vi "LQR_CLEst.vi"() -> ()   [LabVIEW 2019]
uses:
  <vilib>/Analysis/Matrix/Datatypes/RealMatrix.ctl
  <vilib>/Platform/TimedLoop/XDataNode/timing_clust.ctl
  <vilib>/Platform/TimedLoop/XDataNode/nitl_modes.ctl
  <vilib>/Platform/TimedLoop/XDataNode/wakeup.ctl
  <vilib>/Simulation/Shared/_Datatypes/SIM SISO Transfer Function.ctl
  <vilib>/myRIO/Instrument Drivers/Onboard IO/AI/typedefs/AI Reference.ctl
  <vilib>/myRIO/Common/Instrument Driver Framework/Utilities/typedefs/myRIO Generic Hardware Reference.ctl
  <vilib>/myRIO/Common/Instrument Driver Framework/Utilities/typedefs/Hardware Version Enum.ctl
  <vilib>/myRIO/Common/Instrument Driver Framework/Utilities/typedefs/myRIO v1.0 Reference.ctl
  <vilib>/myRIO/Common/Instrument Driver Framework/Utilities/typedefs/Generic FPGA Reference.ctl
  <vilib>/myRIO/Common/Instrument Driver Framework/myRIO v1.0/AI/typedefs/AI Channels List.ctl
  <vilib>/myRIO/Common/Instrument Driver Framework/myRIO v1.0/AI/typedefs/AI Channels Enum.ctl
  <vilib>/myRIO/Common/Instrument Driver Framework/Utilities/typedefs/Analog Scaling Constants List.ctl
  <vilib>/myRIO/Common/Instrument Driver Framework/Utilities/typedefs/Analog Scaling Constants.ctl
  <vilib>/userDefined/High Color/nirio_resource_hc.ctl
  <vilib>/myRIO/Instrument Drivers/Onboard IO/AO/typedefs/AO Reference.ctl
  <vilib>/myRIO/Common/Instrument Driver Framework/myRIO v1.0/AO/typedefs/AO Channels List.ctl
  <vilib>/myRIO/Common/Instrument Driver Framework/myRIO v1.0/AO/typedefs/AO Channels Enum.ctl
  <vilib>/myRIO/Common/Instrument Driver Framework/Utilities/vis/Is FPGA Ref Available.vi
  <vilib>/myRIO/Common/Instrument Driver Framework/myRIO v1.0/AI/vis/myRIO v1.1 Open AI.vi
  <vilib>/myRIO/Instrument Drivers/Onboard IO/AI/vis/Read.vi
  <vilib>/Simulation/DiscreteLinear/Implementation/NILVSim Discrete Transfer Function Direct.llb/SIM Discrete Transfer Function Diagram (SISO).vi
  <vilib>/myRIO/Common/Instrument Driver Framework/myRIO v1.0/AO/vis/myRIO v1.1 Open AO.vi
  <vilib>/myRIO/Instrument Drivers/Onboard IO/AO/vis/Write.vi
  <vilib>/myRIO/Common/Instrument Driver Framework/Utilities/vis/Validate Channels.vi
  <vilib>/myRIO/Common/Instrument Driver Framework/myRIO v1.0/AI/vis/myRIO v1.0 Reserve AI.vi
  <vilib>/Simulation/ContinuousLinear/Implementation/Shared/SIM Transfer Function Support.llb/SIM TransferFunction Normalize to Buffer.vi
  <vilib>/Simulation/DiscreteLinear/Implementation/Shared/SIM Init Discrete States.vi
  <vilib>/Simulation/DiscreteLinear/Implementation/NILVSim Discrete Transfer Function Direct.llb/SIM Transfer Function Direct core (SISO).vi
  <vilib>/myRIO/Common/Instrument Driver Framework/myRIO v1.0/AO/vis/myRIO v1.0 Reserve AO.vi
  <vilib>/myRIO/Common/Instrument Driver Framework/myRIO v1.0/AI/vis/myRIO v1.0 Build MUX Configuration AI.vi
  <vilib>/myRIO/Common/Instrument Driver Framework/myRIO v1.0/Resource Manager/vis/myRIO v1.0 Reserve Channel List.vi
  <vilib>/Simulation/ContinuousLinear/Implementation/Shared/SIM Transfer Function Support.llb/SIM TransferFunction Normalize.vi
  <vilib>/myRIO/Common/Instrument Driver Framework/myRIO v1.0/AO/vis/myRIO v1.0 Build MUX Configuration AO.vi
  <vilib>/myRIO/Common/Instrument Driver Framework/myRIO v1.0/Resource Manager/vis/myRIO v1.0 Reserve Channel.vi
  <vilib>/myRIO/Common/Instrument Driver Framework/myRIO v1.0/Resource Manager/vis/myRIO v1.0 Unreserve Channel.vi
  <vilib>/Simulation/Implementation/Shared/SIM Polynomials.llb/SIM Remove Zero Coefficients (DBL).vi
  <vilib>/myRIO/Common/Instrument Driver Framework/myRIO v1.0/Resource Manager/vis/myRIO v1.0 Build Mutex Name.vi
  <vilib>/Simulation/Implementation/Shared/SIM Polynomials.llb/SIM Divide Polynomials (DBL).vi
  <vilib>/Simulation/Implementation/Shared/SIM BuildSimErr.vi
  <vilib>/Utility/VariantDataType/GetNumericInfo.vi
  <vilib>/Utility/error.llb/Error Cluster From Error Code.vi
  <vilib>/myRIO/Common/Instrument Driver Framework/myRIO v1.0/myRIO v1.1 Open.vi
  <vilib>/myRIO/Common/Instrument Driver Framework/myRIO v1.0/AI/vis/myRIO v1.0 Get Scaling Constants AI.vi
  <vilib>/myRIO/Common/Instrument Driver Framework/Utilities/vis/IO Manager.vi
  <vilib>/myRIO/Common/Instrument Driver Framework/Utilities/vis/Configuration Manager.vi
  <vilib>/myRIO/Common/Instrument Driver Framework/myRIO v1.0/myRIO v1.0 Close.vi
  <vilib>/myRIO/Common/Instrument Driver Framework/myRIO v1.0/AI/vis/myRIO v1.0 Read AI.vi
  <vilib>/myRIO/Common/Instrument Driver Framework/myRIO v1.0/AO/vis/myRIO v1.0 Get Scaling Constants AO.vi
  <vilib>/myRIO/Common/Instrument Driver Framework/myRIO v1.0/AO/vis/myRIO v1.0 Write AO.vi
  <vilib>/Analysis/Matrix/Numeric/Multiply/Multiply - RM,RM.vi
  <vilib>/Analysis/Matrix/Numeric/Subtract/Subtract (Elementwise) - R,RM.vi
  <vilib>/Analysis/Matrix/Numeric/Multiply/Multiply - RM,R.vi
  <vilib>/Analysis/Matrix/Numeric/Add/Add - RM,RM.vi
  <vilib>/platform/TimedLoop/XDataNode/XDataNode.xnode
  <vilib>/Simulation/Implementation/XNodeFramework/SimXNode/SimX.xnode
  <vilib>/myRIO/Express VI/Onboard IO/AI/AI Express VI.xnode
  <vilib>/myRIO/Instrument Drivers/Onboard IO/AI/vis/myRIO AI Open.xnode
  <vilib>/myRIO/Express VI/Onboard IO/AO/AO Express VI.xnode
  <vilib>/myRIO/Instrument Drivers/Onboard IO/AO/vis/myRIO AO Open.xnode
  <vilib>/Platform/TimedLoop/XDataNode/XDNodeRunTimeDep.lvlib
  <vilib>/myRIO/Instrument Drivers/Onboard IO/AI/AI.lvlib
  <vilib>/myRIO/Instrument Drivers/Onboard IO/AO/AO.lvlib
  <vilib>/ptbypt/NI_PtbyPt.lvlib
  <vilib>/Analysis/Matrix/NI_Matrix.lvlib
panel:
  in  "amplitude":dbl=1.0 format="%0.2f"
  out "Impulse Pattern":dbl(graph)
  out "output y(k)":dbl=6.43996164946016e-05
  in  "D":dbl=7.3
  in  "P":dbl=5291.0
  out "x*y":dbl(graph)=-8.32082689025263
  in  "C":T1=[[1.0, 0.0]]
  out "transposed matrix":T1=[[7.6247197208905344e-06], [0.00010412510161981911]]
  in  "B":T1=[[0.0], [17.2685]]
  in  "A":T1=[[0.0, 1.0], [-5529.8, -0.5327]]
  in  "L":T1=[[2200.0], [1953300.0]]
  in  "stopNoise":bool=TRUE
  in  "gain_noise":dbl=0.2
  out "uniform white noise":dbl(graph)=-0.031193239239623867
  in  "AmpWhitehNoise":dbl=1.0 format="%0.2f"
  out "Iteration Duration":i64(graph)=347
  in  "Max FRF current 0-1000mA":dbl=4.0
  in  "Stop FRF":bool=TRUE
  in  "esc":bool
  out "x[um]":cluster{dbl, dbl, dbl, dbl, dbl}(graph)={-8.303163599999976, 0.03990822535355048, -0.0, -8.32082689025263, 946.4168275057085}
  out "Current Output EM":dbl(graph)=0.03990822535355048
  in  "Stop EM + FRF":bool=TRUE
  out "left[V]":dbl=-0.0
  out "right[V]":dbl=-0.0
  out "um":dbl=376.9531636
  # "mA"
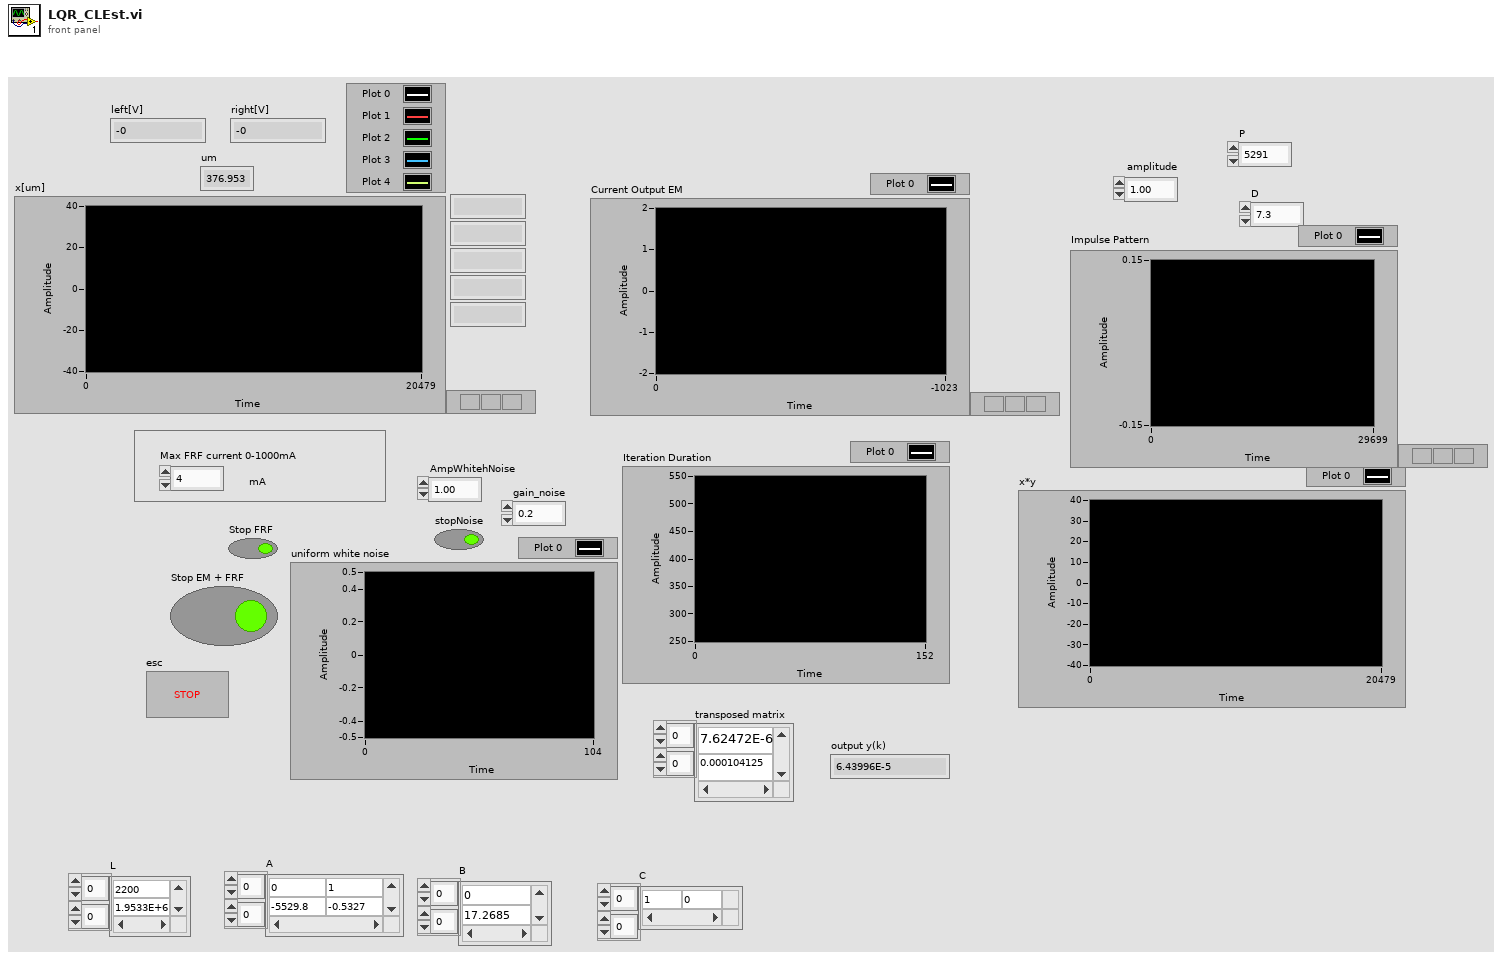
[diagram p1: front panel]
types:
  T1 = typedef "NI_Matrix.lvlib/RealMatrix.ctl" = dbl[][]
  T2 = typedef "XDNodeRunTimeDep.lvlib/timing_clust.ctl" = cluster{"Expected End [f-1]":u64, "Actual End [f-1]":u64, "Finished Late? [f-1]":bool, "Expected End [i-1]":u64, "Actual End [i-1]":u64, "Finished Late? [i-1]":bool, "Expected Start [i]":u64, "Actual Start [i]":u64, "Expected Start [f]":u64, "Actual Start [f]":u64, "Source Name":string, "Structure Name":string, "Period":i64, "Deadline":i64, "Offset":i64, "Start":i64, "Priority":i32, "Timeout":i32, "Mode":T3, "Wakeup Reason":T4, "Error":errorcluster, "Source Type":string, "Secondary Source Type":string, "Global End Time":u64, "Global Start Time":u64, "Frame Duration":u64, "Iteration Duration":u64, "Assigned CPU":i32, "I/O Scan Engine Mode":u32}
  T3 = typedef "XDNodeRunTimeDep.lvlib/nitl_modes.ctl" = enum32{"No Change", "Process missed periods, maintain original phase", "Discard missed periods, maintain original phase", "Process missed periods, ignore original phase", "Discard missed periods, ignore original phase"}
  T4 = typedef "XDNodeRunTimeDep.lvlib/wakeup.ctl" = enum32{"Normal", "Aborted", "Asynchronous wakeup", "Timing source error", "Timed loop error", "Timeout"}
  T5 = typedef "SIM SISO Transfer Function.ctl" = cluster{"Numerator":dbl[], "Denominator":dbl[]}
  T6 = typedef "AI.lvlib/AI Reference.ctl" = cluster{"myRIO Reference":T7, "AI Channels List":T11, "AI Scaling Constants List":T13}
  T7 = typedef "myRIO Generic Hardware Reference.ctl" = cluster{"myRIO Model":T8, "myRIO Hardware Reference":T9}
  T8 = typedef "Hardware Version Enum.ctl" = enum16{"Unknown", "myRIO-1900", "myRIO-1950", "roboRIO", "NI ELVIS RIO CM", "ELVIS III"}
  T9 = typedef "myRIO v1.0 Reference.ctl" = cluster{"Generic FPGA Reference":T10, "Allow multiple opens":bool}
  T10 = typedef "Generic FPGA Reference.ctl" = refnum<k20>
  T11 = typedef "AI Channels List.ctl" = T12[]
  T12 = typedef "AI Channels Enum.ctl" = enum16{"Not Connected", "AudioIn/Left", "AudioIn/Right", "C/AI0", "C/AI1", "A/AI0", "A/AI1", "A/AI2", "A/AI3", "A/AI4", "A/AI5", "A/AI6", "A/AI7", "B/AI0", "B/AI1", "B/AI2", "B/AI3", "B/AI4", "B/AI5", "B/AI6", "B/AI7", "AI/AI0", "AI/AI1", "AI/AI2", "AI/AI3", "A/AI0 (DIFF)", "A/AI1 (DIFF)", "A/AI2 (DIFF)", "A/AI3 (DIFF)", "B/AI0 (DIFF)", "B/AI1 (DIFF)", "B/AI2 (DIFF)", "B/AI3 (DIFF)"}
  T13 = typedef "Analog Scaling Constants List.ctl" = T14[]
  T14 = typedef "Analog Scaling Constants.ctl" = cluster{"LSB Weight (Volts)":dbl, "Offset (Volts)":dbl, "Signed?":bool}
  T15 = typedef "nirio_resource_hc.ctl" = tag
  T16 = typedef "AO.lvlib/AO Reference.ctl" = cluster{"myRIO Reference":T7, "AO Channel List":T17, "AO Scaling Constant List":T13}
  T17 = typedef "AO Channels List.ctl" = T18[]
  T18 = typedef "AO Channels Enum.ctl" = enum16{"Not Connected", "AudioOut/Left", "AudioOut/Right", "C/AO0", "C/AO1", "A/AO0", "A/AO1", "B/AO0", "B/AO1"}
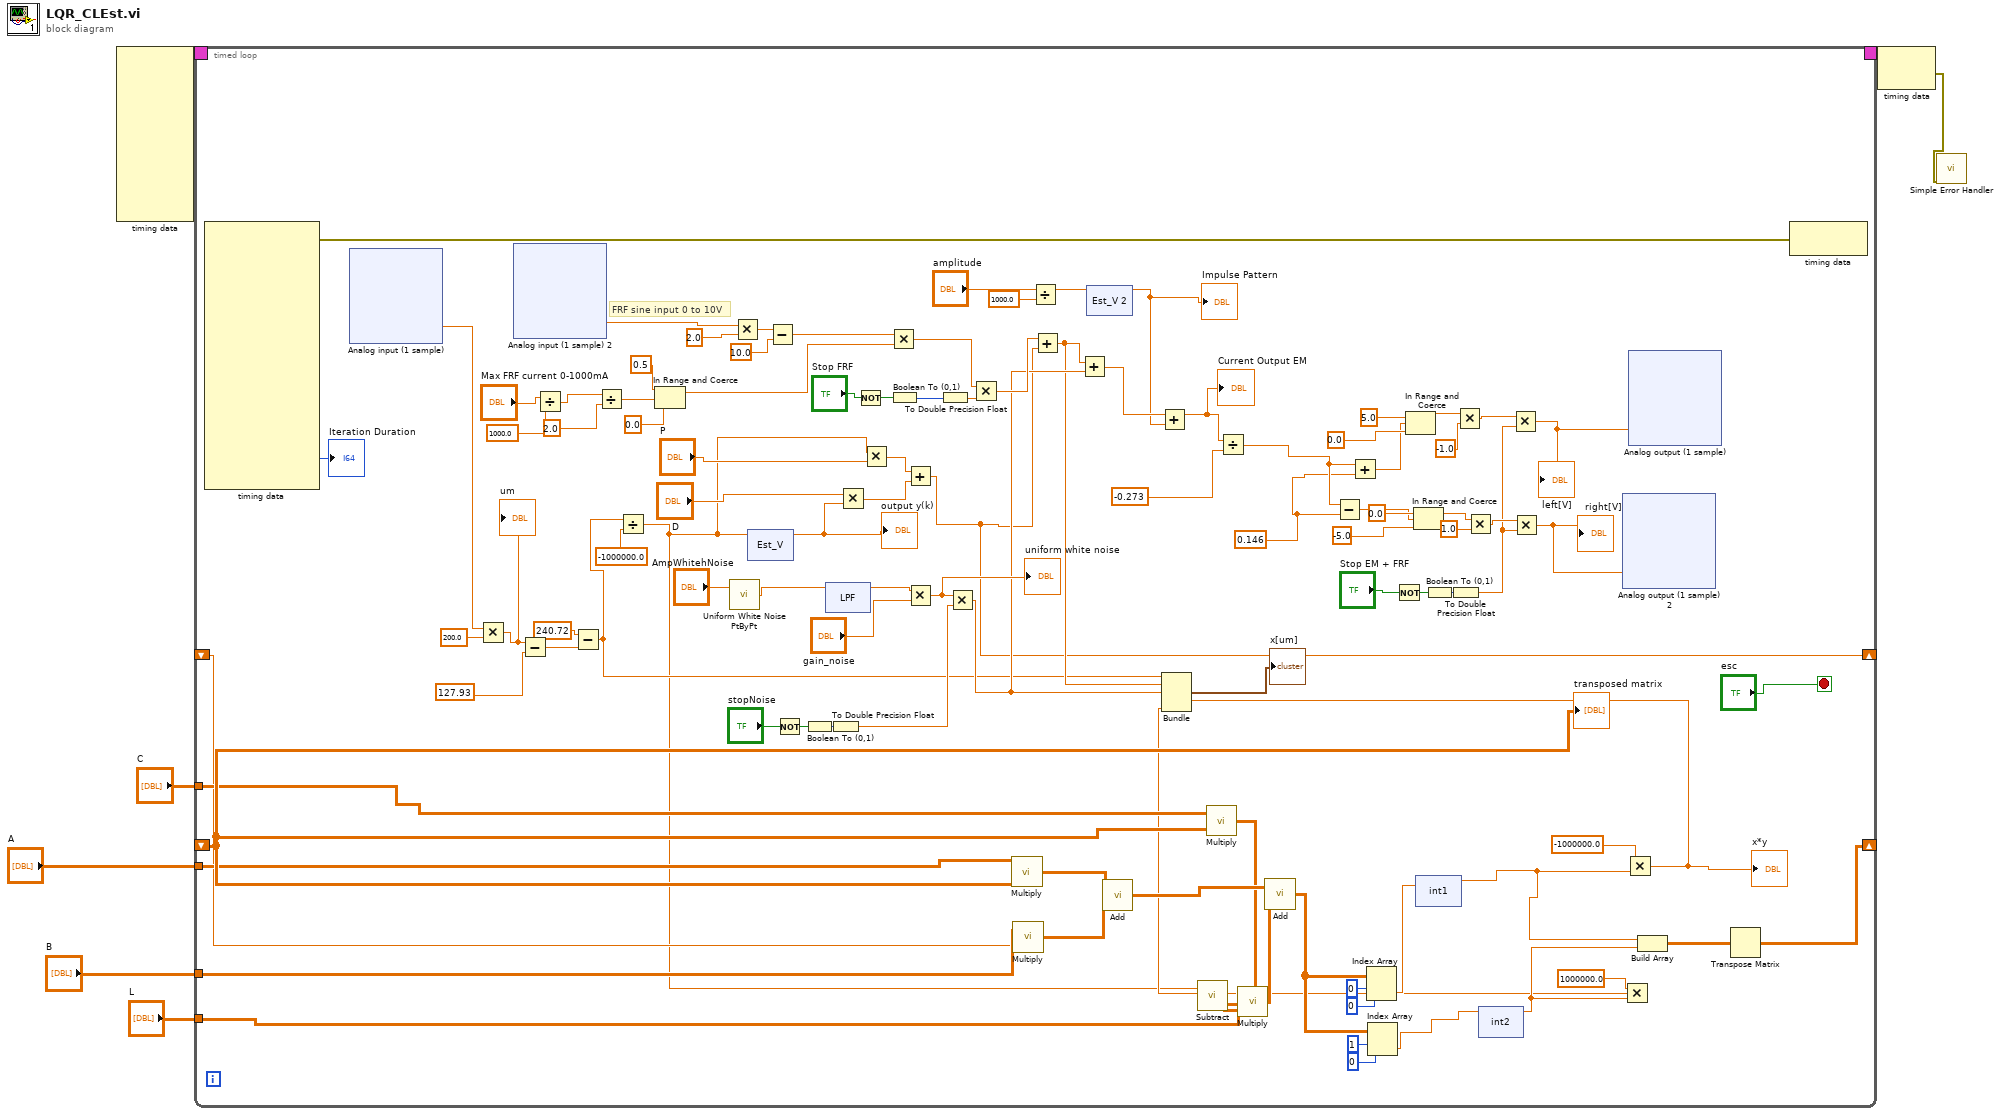
[diagram p0: block diagram]
diagram:
  n1 = node-c288() -> (w7:T2)  [unwired: 10 in]
  n2 = timed-loop {
    timing: w7 -> [_]
    timing-out: [_] -> w6
    shift-right: [w35] -> _
    shift-left: _ -> [w36]
    tunnel: "A" -> [w32]
    tunnel: "B" -> [w31]
    tunnel: "C" -> [w30]
    tunnel: "L" -> [w29]
    shift-right: [w21] -> _
    shift-left: _ -> [w26]
    stop <- "esc" stop-if-true
    w69 = 0.146 ("y")
    # "FRF sine input 0 to 10V"
    n3 = node-c288() -> (w110:errorcluster, →"Iteration Duration":i64)  [unwired: 1 in, 15 out]
    n4 = xnode "Analog input (1 sample)"() -> ("C/AI1 (AI1)"=w65:dbl)  [unwired: 1 in, 1 out]
    n5 = Multiply(x=w65, y=200.0) -> (x*y=w108:dbl)
    "um" <- w108
    n6 = xnode "Analog input (1 sample) 2"() -> ("C/AI0 (AI0)"=w87:dbl)  [unwired: 1 in, 1 out]
    n7 = Subtract(x=w108, y=127.93) -> (x-y=w107:dbl)
    n8 = Divide(x="Max FRF current 0-1000mA", y=1000.0) -> (x/y=w76:dbl)
    n9 = Subtract(x=240.72, y=w107) -> (x-y=w48:dbl)
    n10 = Divide(x=w76, y=2.0) -> (x/y=w80:dbl)
    n11 = Divide(x=w48, y=-1000000.0) -> (x/y=w14:dbl)
    n12 = In Range and Coerce(upper limit=0.5, x=w80, lower limit=0.0) -> (coerced(x)=w77:dbl)  [unwired: 1 out]
    n13 = call <vilib>:"Uniform White Noise PtByPt.vi"("amplitude"="AmpWhitehNoise") -> ("uniform white noise"=w58:dbl)  [unwired: 2 in]
    n14 = Multiply(x=w87, y=2.0) -> (x*y=w85:dbl)
    n15 = xnode "Est_V"("input u(k)"=w14) -> ("output y(k)"=w16:dbl)  [unwired: 2 in, 1 out]
    "output y(k)" <- w16
    n16 = Subtract(x=w85, y=10.0) -> (x-y=w82:dbl)
    n17 = Not(x="stopNoise") -> (.not. x?=w56:bool)
    n18 = Boolean To (0,1)(Boolean=w56) -> (0, 1=w57:i16)
    n19 = xnode "LPF"("input u(k)"=w58) -> ("output y(k)"=w55:dbl)  [unwired: 2 in, 1 out]
    n20 = To Double Precision Float(number=w57) -> (double precision float=w52:dbl)
    n21 = Multiply(x="D", y=w16) -> (x*y=w27:dbl)
    n22 = Not(x="Stop FRF") -> (.not. x?=w90:bool)
    n23 = Multiply(x=w14, y="P") -> (x*y=w28:dbl)
    n24 = Multiply(x=w82, y=w77) -> (x*y=w83:dbl)
    n25 = Boolean To (0,1)(Boolean=w90) -> (0, 1=w89:i16)
    n26 = Add(x=w28, y=w27) -> (x+y=w21:dbl)
    n27 = Multiply(x=w55, y="gain_noise") -> (x*y=w51:dbl)
    "uniform white noise" <- w51
    n28 = To Double Precision Float(number=w89) -> (double precision float=w88:dbl)
    n29 = Multiply(x=w51, y=w52) -> (x*y=w50:dbl)
    n30 = Multiply(x=w83, y=w88) -> (x*y=w92:dbl)
    n31 = call-poly <vilib>:"Multiply.vi"("Real Matrix B"=w36, "Real Matrix A"=w32) -> ("A * B"=w47:T1)
    n32 = call-poly <vilib>:"Multiply.vi"("Real Scalar c"=w26, "Real Matrix A"=w31) -> ("A * c"=w46:T1)
    n33 = Divide(x="amplitude", y=1000.0) -> (x/y=w11:dbl)
    n34 = Add(x=w92, y=w21) -> (x+y=w49:dbl)
    n35 = Add(x=w49, y=w50) -> (x+y=w13:dbl)
    n36 = xnode "Est_V 2"("input u(k)"=w11) -> ("output y(k)"=w8:dbl)  [unwired: 2 in, 1 out]
    "Impulse Pattern" <- w8
    n37 = call-poly <vilib>:"Add.vi"("Real Matrix B"=w46, "Real Matrix A"=w47) -> ("A + B"=w45:T1)
    n38 = Add(x=w13, y=w8) -> (x+y=w9:dbl)
    "Current Output EM" <- w9
    n39 = call-poly <vilib>:"Multiply.vi"("Real Matrix B"=w36, "Real Matrix A"=w30) -> ("A * B"=w34:T1)
    n40 = call-poly <vilib>:"Subtract.vi"("Real Matrix A"=w34, "Real Scalar c"=w14) -> ("c - A"=w38:T1)
    n41 = Divide(x=w9, y=-0.273) -> (x/y=w70:dbl)
    n42 = call-poly <vilib>:"Multiply.vi"("Real Matrix B"=w38, "Real Matrix A"=w29) -> ("A * B"=w44:T1)
    n43 = call-poly <vilib>:"Add.vi"("Real Matrix B"=w44, "Real Matrix A"=w45) -> ("A + B"=w39:T1)
    n44 = Subtract(x=w70, y=w69) -> (x-y=w71:dbl)
    n45 = Add(x=w70, y=w69) -> (x+y=w72:dbl)
    n46 = Index Array(array=w39, index (row)=0, index (col)=0 ("disabled index (col)")) -> (element=w23:dbl)
    n47 = Index Array(array=w39, index (row)=1, index (col)=0 ("disabled index (col)")) -> (element=w22:dbl)
    n48 = Not(x="Stop EM + FRF") -> (.not. x?=w95:bool)
    n49 = In Range and Coerce(upper limit=5.0 ("x"), x=w72, lower limit=0.0) -> (coerced(x)=w62:dbl)  [unwired: 1 out]
    n50 = In Range and Coerce(upper limit=0.0 ("x"), x=w71, lower limit=-5.0) -> (coerced(x)=w100:dbl)  [unwired: 1 out]
    n51 = xnode "int1"("input u(k)"=w23) -> ("output y(k)"=w15:dbl)  [unwired: 2 in, 1 out]
    n52 = Boolean To (0,1)(Boolean=w95) -> (0, 1=w97:i16)
    n53 = To Double Precision Float(number=w97) -> (double precision float=w66:dbl)
    n54 = Multiply(x=w62, y=-1.0) -> (x*y=w68:dbl)
    n55 = Multiply(x=w100, y=1.0) -> (x*y=w67:dbl)
    n56 = xnode "int2"("input u(k)"=w22) -> ("output y(k)"=w19:dbl)  [unwired: 2 in, 1 out]
    n57 = Multiply(x=w68, y=w66) -> (x*y=w64:dbl)
    "left[V]" <- w64
    n58 = Multiply(x=w67, y=w66) -> (x*y=w63:dbl)
    "right[V]" <- w63
    n59 = Multiply ("Multiply.vi")(x=1000000.0 ("y"), y=w19) -> (x*y=w17:dbl)
    n60 = xnode "Analog output (1 sample) 2"("C/AO1 (AO1)"=w63) -> ()  [unwired: 1 in, 1 out]
    n61 = Multiply ("Multiply.vi")(x=-1000000.0 ("y"), y=w15) -> (x*y=w20:dbl)
    "x*y" <- w20
    n62 = Bundle(w48, w49, w50, w20, w17) -> (→"x[um]":cluster{dbl, dbl, dbl, dbl, dbl})  [unwired: 1 in]
    n63 = xnode "Analog output (1 sample)"("C/AO0 (AO0)"=w64) -> ()  [unwired: 1 in, 1 out]
    n64 = Build Array(w15, w19) -> (w37:T1)
    n65 = Transpose Matrix(1:w37) -> (0:w35:T1)
    n66 = node-c288(w110) -> ()  [unwired: 1 out]
    "transposed matrix" <- w36
  }
  n67 = node-c288(w6) -> (w5:errorcluster)
  n68 = call <vilib>:"Simple Error Handler.vi"("error in (no error)"=w5) -> ()  [unwired: 4 in, 5 out]
